vi "Frequency ACQ.vi"(8 "error in (no error)":errorcluster, 10 "Frequency":dbl, 11 "ACQ Generador in":refnum<class "ACQ Generador.lvclass">) -> (0 "error out":errorcluster, 3 "ACQ Generador out":refnum<class "ACQ Generador.lvclass">)   [LabVIEW 2020, in "ACQ Generador.lvlib" / "ACQ Generador.lvclass"]
uses:
  ACQ Generador.lvclass
  ACQ Generador.lvclass/ACQ Generador.ctl
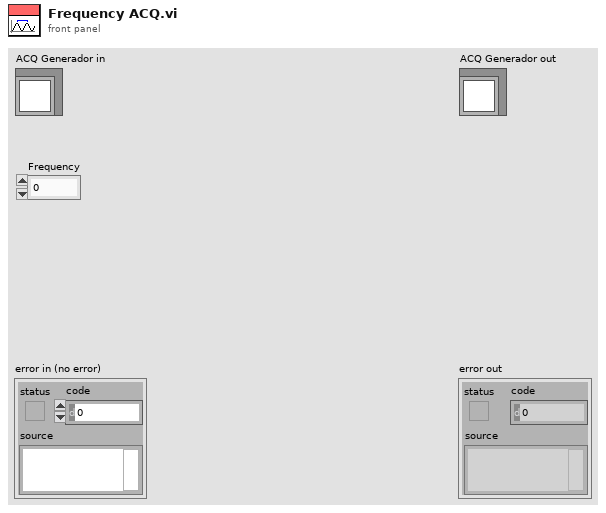
[diagram p1: front panel]
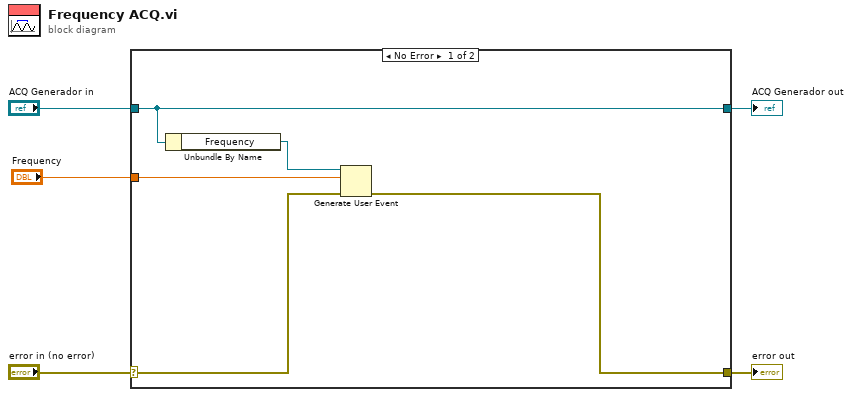
[diagram p0: block diagram]
diagram:
  n1 = case shown="No Error" "error in (no error)" {
    selector: "error in (no error)" -> [w7 w12]
    tunnel: [w6 w12] -> w4
    tunnel: [w10 w11] -> w2
    tunnel: "ACQ Generador in" -> [w10 w11]
    tunnel: "Frequency" -> [w9 _]
    frame No Error {
      n2 = Unbundle By Name(w10) -> ("Frequency"=w8:refnum<user-event>)
      n3 = Generate User Event(user event=w8, event data cluster=w9, error in=w7) -> (error out=w6:errorcluster)  [unwired: 1 in, 1 out]
    }
    frame Error {
    }
  }
  "error out" <- w4
  "ACQ Generador out" <- w2
